vi "closeCheck_fw103.vi"(8 "Close":bool, 9 "Device reference input":refnum<k24>) -> (1 "error out":errorcluster)   [LabVIEW 2020]
uses:
  C:/Users/OPMuser/Documents/labview/fw103/Thorlabs.MotionControl.Controls.dll
  Thorlabs.MotionControl.Controls.dll
  <vilib>/ErrorRing/Error Ring.xnode
panel:
  out "Wheel on":bool
  # "Supply with a boolean input, if it is true it will close the device, otherwise it does nothing"
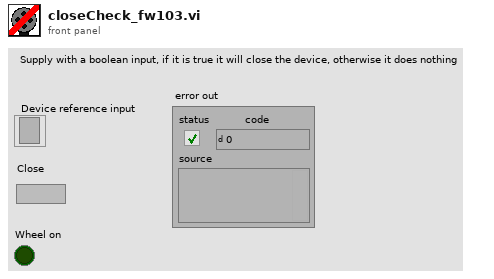
[diagram p1: front panel]
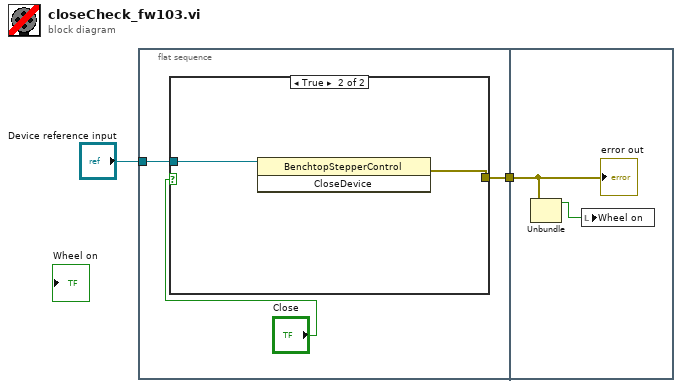
[diagram p0: block diagram]
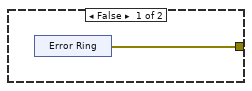
[diagram p2: hidden frame]
diagram:
  n1 = flat-sequence {
    tunnel: "Device reference input" -> [w5]
    tunnel: [w4] -> w1
    tunnel: w1 -> [w10]
    frame #0 {
      n2 = case shown="True" "Close" {
        tunnel: w5 -> [_ w9]
        tunnel: [w6 w8] -> w4
        frame False {
          n3 = xnode "Error Ring"() -> ("error out"=w6:errorcluster)
        }
        frame True {
          n4 = invoke class="BenchtopStepperControl" method="CloseDevice"(reference=w9) -> (error out=w8:errorcluster)  [unwired: 2 in, 2 out]
        }
      }
    }
    frame #1 {
      n5 = Unbundle(w10) -> ("status"=w11:bool)  [unwired: 2 out]
      n6 = local write "Wheel on"(w11) -> ()
      "error out" <- w10
    }
  }
